vi "Predefinied Event.vi"   [LabVIEW 2019, in "Event.lvclass"]
uses:
  Event.lvclass
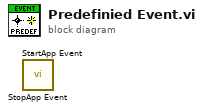
[diagram p0: block diagram]
diagram:
  n1 = call "StopApp Event.vi"() -> ()  [unwired: 10 in, 2 out]
  n2 = call "StartApp Event.vi"() -> ()  [unwired: 10 in, 2 out]
